vi "Get S-Param Names - SParam.vi"(11 "Array in":refnum<vi>) -> (3 "Plot Names":string[](array[string]))   [LabVIEW 2023, in "FPT_SParam UI.lvlib"]
uses:
  FPT_SParam UI.lvlib
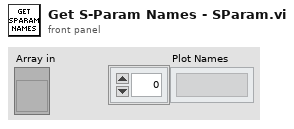
[diagram p1: front panel]
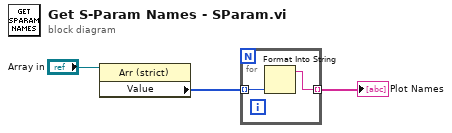
[diagram p0: block diagram]
diagram:
  n1 = property on="Property Node" class="Arr (strict)"(reference="Array in") -> ("Value"=w3:enum16{"S11", "S21", "S12", "S22"}[])  [unwired: 1 in, 2 out]
  n2 = for {
    tunnel: w3 -> [w4] mode=indexing
    tunnel: [w5] -> w2 mode=indexing
    n3 = Format Into String(w4) -> (resulting string=w5:string)  [unwired: 3 in, 1 out]
  }
  "Plot Names" <- w2
